vi "setServiceMode.vi"(8 "error in (no error)":errorcluster, 10 "ServiceMode":bool, 11 "ISA010 in":refnum<class "ISA010.lvclass">) -> (0 "error out":errorcluster, 3 "ISA010 out":refnum<class "ISA010.lvclass">)   [LabVIEW 2017, in "ISA010.lvlib" / "ISA010.lvclass"]
uses:
  ISA010.lvclass
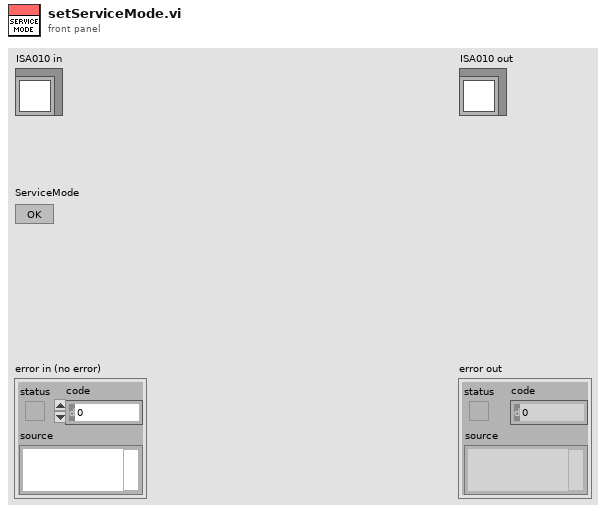
[diagram p1: front panel]
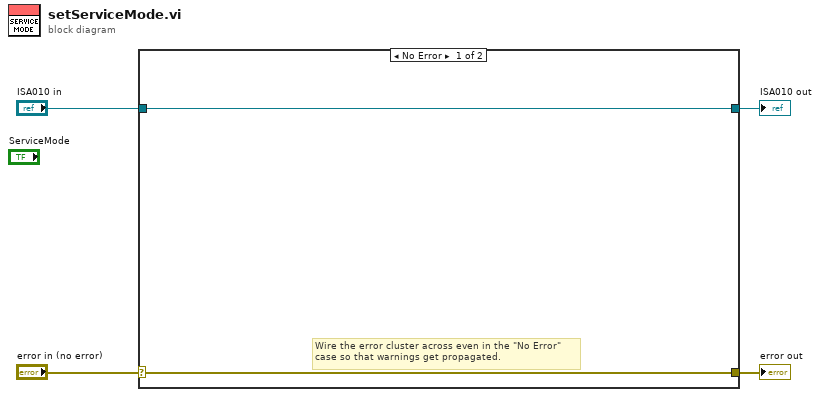
[diagram p0: block diagram]
diagram:
  n1 = case shown="No Error" "error in (no error)" {
    selector: "error in (no error)" -> [w5 w8]
    tunnel: [w5 w8] -> w3
    tunnel: [w6 w7] -> w1
    tunnel: "ISA010 in" -> [w6 w7]
    frame No Error {
      # "Wire the error cluster across even in the \"No Error\"\ncase so that warnings get propagated."
    }
    frame Error {
    }
  }
  "error out" <- w3
  "ISA010 out" <- w1
